vi "CL3IF_AutoZeroGroup.vi"(7 "group":T1 items=["GROUP1"=1, "GROUP2"=2], 8 "error in":errorcluster {"code" format="%x"}, 10 "onOff":bool, 11 "deviceId":i32) -> (0 "error out":errorcluster {"code" format="%x"})   [LabVIEW 2020, in "Keyence CL-3000.lvlib"]
doc: "This function turns auto zero on/off for the OUT group set with terminal allocation."
uses:
  Keyence CL-3000.lvlib
  enums/CL3IF_ZERO_GROUP.ctl
  Private/enums/Function Name.ctl
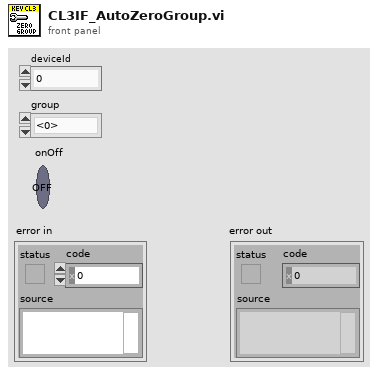
[diagram p1: front panel]
types:
  T1 = typedef "Keyence CL-3000.lvlib/CL3IF_ZERO_GROUP.ctl" = u16
  T2 = typedef "Keyence CL-3000.lvlib/Function Name.ctl" = enum16{"Initialize", "Close", "CL3IF_GetMeasurementData", "CL3IF_GetTrendIndex", "CL3IF_GetTrendData", "CL3IF_GetStorageIndex", "CL3IF_GetStorageData", "CL3IF_AutoZeroMulti", "CL3IF_AutoZeroGroup", "CL3IF_TimingMulti", "CL3IF_TimingGroup", "CL3IF_ResetMulti", "CL3IF_ResetGroup", "CL3IF_LightControl", "CL3IF_MeasurementControl", "CL3IF_SwitchProgram", "CL3IF_GetProgramNo", "CL3IF_StartStorage", "CL3IF_StopStorage", "CL3IF_ClearStorageData", "CL3IF_GetPulseCount", "CL3IF_ResetPulseCount", "CL3IF_GetLightWaveform"}
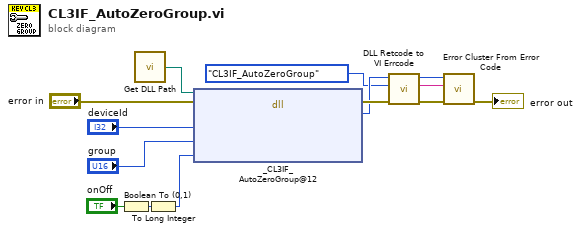
[diagram p0: block diagram]
diagram:
  n1 = Boolean To (0,1)(Boolean="onOff") -> (0, 1=w10:i16)
  n2 = call "Get DLL Path.vi"() -> ("DLL Path"=w9:path)  [unwired: 1 in]
  n3 = To Long Integer(number=w10) -> (32bit integer=w5:i32)
  n4 = dll-call lib="C:/Program Files (x86)/National Instruments/LabVIEW 2018/instr.lib/Keyence CL-3000/CL3_IF.dll" fn="_CL3IF_AutoZeroGroup@12"(path in=w9, error in="error in", "deviceId"="deviceId", "group"="group", "onOff"=w5) -> (error out=w4:errorcluster, "RC"=w3:i32)  [unwired: 4 in, 1 out]
  n5 = call "DLL Retcode to VI Errcode.vi"("error in (no error)"=w4, "Function Name"=Function_Name."CL3IF_AutoZeroGroup", "DLL Retcode"=w3) -> ("error out"=w14:errorcluster, "ErrorMessage"=w2:string, "VI Errcode"=w13:i32)  [unwired: 6 in]
  n6 = call <vilib>:"Error Cluster From Error Code.vi"("error in (no error)"=w14, "error message (\"\")"=w2, "error code (0)"=w13) -> ("error out"=→"error out":errorcluster)  [unwired: 6 in]
